vi "Add Song To Queue.vi"(8 "error in (no error)":errorcluster, 10 "Song":refnum<class "Song.lvclass">, 11 "SongQueueActor In":refnum<class "SongQueueActor.lvclass">) -> (0 "error out":errorcluster, 3 "SongQueueActor Out":refnum<class "SongQueueActor.lvclass">)   [LabVIEW 2015, in "SongQueueActor.lvlib" / "SongQueueActor.lvclass"]
uses:
  SongQueueActor.lvclass
  file/MusicElement/Song/Song.lvclass
  SongQueueActor.lvclass/SongQueueActor.ctl
  controls/Queue Song Display.ctl
  file/MusicElement/Song/Song Duration.ctl
  controls/Dequeue Control.ctl
  builds/xctls/Song Queue/Song Queue.lvlibp/app/xctls/SongQueue/Song Queue.xctl
  file/MusicElement/MusicElementLibrary/MusicElementLibrary.lvclass
  SongPlayerActor/SongPlayerActor Messages/Play Song Msg/Play Song Msg.lvclass
  AlbumImageActor/AlbumImageActor Messages/Download Album Image Msg/Download Album Image Msg.lvclass
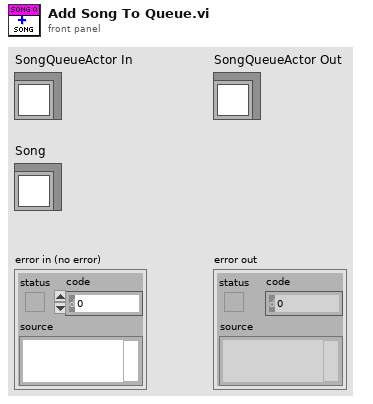
[diagram p1: front panel]
types:
  T1 = typedef "Queue Song Display.ctl" = cluster{"Song Name":string, "Artist":string, "Album":string, "Duration (s)":T2, "UID":string, "Dequeue":T3}
  T2 = typedef "Song.lvclass/Song Duration.ctl" = timestamp
  T3 = typedef "Dequeue Control.ctl" = bool
  T4 = typedef "Song Queue.lvlibp/Queue Song Display.ctl" = cluster{"Song Name":string, "Artist":string, "Album":string, "Duration (s)":T5, "UID":string, "Dequeue":T6}
  T5 = typedef "Song Queue.lvlibp/Song.lvclass/Song Duration.ctl" = timestamp
  T6 = typedef "Song Queue.lvlibp/Dequeue Control.ctl" = bool
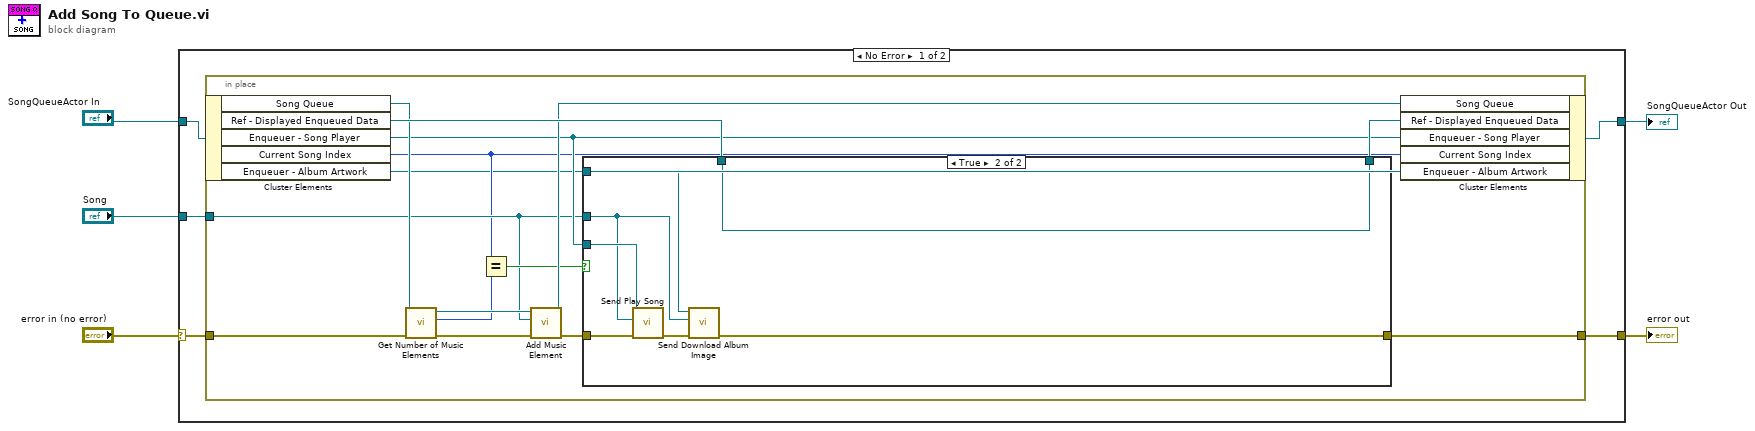
[diagram p0: block diagram]
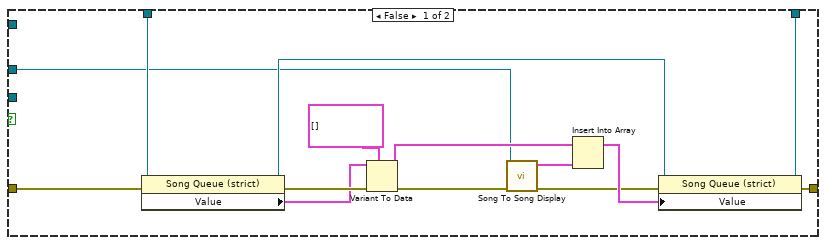
[diagram p2: hidden frame]
diagram:
  n1 = case shown="No Error" "error in (no error)" {
    selector: "error in (no error)" -> [w8 w48]
    tunnel: [w6 w48] -> w4
    tunnel: [w7 w47] -> w3
    tunnel: "SongQueueActor In" -> [w9 w47]
    tunnel: "Song" -> [w10 _]
    frame No Error {
      n2 = in-place {
        in-place-border: w10 -> [w13]
        in-place-border: w8 -> [w20]
        in-place-border: [w24] -> w6
        n3 = in-place-cluster #1(w9) -> ("Song Queue"=w19:refnum<class "SongLibrary.lvclass">, "Ref - Displayed Enqueued Data"=w25:refnum<vi>, "Enqueuer - Song Player"=w15:refnum<class "Message Enqueuer.lvclass">, "Current Song Index"=w12:i32, "Enqueuer - Album Artwork"=w11:refnum<class "Message Enqueuer.lvclass">)
        n4 = call "Get Number of Music Elements.vi"("error in (no error)"=w20, "MusicElementLibrary in"=w19) -> ("error out"=w21:errorcluster, "Size"=w17:i32, "MusicElementLibrary out"=w18:refnum<class "SongLibrary.lvclass">)  [unwired: 7 in]
        n5 = Equal?(x=w12, y=w17) -> (x = y?=w16:bool)
        n6 = call "Add Music Element.vi"("error in (no error)"=w21, "MusicElement"=w13, "MusicElementLibrary in"=w18) -> ("error out"=w14:errorcluster, "MusicElementLibrary out"=w22:refnum<class "SongLibrary.lvclass">)  [unwired: 7 in]
        n7 = case shown="True" w16 {
          tunnel: w25 -> [w39 w46]
          tunnel: [w34 w40] -> w24
          tunnel: [w33 w46] -> w23
          tunnel: w13 -> [w27 w41]
          tunnel: w15 -> [_ w44]
          tunnel: w14 -> [w26 w45]
          tunnel: w11 -> [_ w42]
          frame False {
            n8 = property class="Song Queue (strict)"(reference=w39, error in=w26) -> (reference out=w28:refnum<vi>, error out=w38:errorcluster, "Value"=w37:T4[])
            n9 = Variant To Data(error in=w38, type=T1[] [], Variant=w37) -> (data=w32:T1[], error out=w35:errorcluster)
            n10 = call "Song To Song Display.vi"("error in (no error)"=w35, "Song"=w27) -> ("error out"=w29:errorcluster, "Song DIsplay"=w31:T1)  [unwired: 8 in]
            n11 = Insert Into Array(array=w32, new element=w31) -> (w30:T1[])  [unwired: 1 in]
            n12 = property class="Song Queue (strict)"(reference=w28, error in=w29, "Value"=w30) -> (reference out=w33:refnum<vi>, error out=w34:errorcluster)
          }
          frame True {
            n13 = call "Send Play Song.vi"("error in (no error)"=w45, "Song"=w41, "Message Enqueuer in"=w44) -> ("error out"=w43:errorcluster)  [unwired: 7 in, 1 out]
            n14 = call "Send Download Album Image.vi"("error in (no error)"=w43, "Song"=w41, "Message Enqueuer in"=w42) -> ("error out"=w40:errorcluster)  [unwired: 7 in, 1 out]
          }
        }
        n15 = in-place-cluster #1("Song Queue"=w22, "Ref - Displayed Enqueued Data"=w23, "Enqueuer - Song Player"=w15, "Current Song Index"=w12, "Enqueuer - Album Artwork"=w11) -> (w7:refnum<class "SongQueueActor.lvclass">)
      }
    }
    frame Error {
    }
  }
  "error out" <- w4
  "SongQueueActor Out" <- w3
